vi "Kaelus PIM Set Stimulus.vi"(4 "Force? (f)":bool, 6 "Legacy (f)?":bool, 7 "TestSetDef":T1={"General"={"ID"=0, "Model"="", "Dual Port?"=FALSE, "Options"="", "Options"={"E"=FALSE, "K"=FALSE, "H"=FALSE, "W"=FALSE, "F"=FALSE}, "Cal File"=path ""}, "Receiver"={"Fstart, MHz"=0.0, "Fstop MHz"=0.0, "Fstep MHz"=0.0, "IF, MHz"=0.0}, "RX Band"={"Fstart, MHz"=0.0, "Fstop MHz"=0.0}, "TX 1"={"Fstart, MHz"=0.0, "Fstop MHz"=0.0, "Pmax, dBm"=0.0, "Pstep, dB"=0.0}, "TX 2"={"Fstart, MHz"=0.0, "Fstop MHz"=0.0, "Pmax, dBm"=0.0, "Pstep, dB"=0.0}, "Low-side?"=TRUE}, 8 "error in (no error)":errorcluster, 11 "Stimulus":T2={"Carrier Frequencies"={"C1 Freq, MHz"=0.0, "C2 Freq, MHz"=0.0}, "Carrier Powers"={"C1 Power,dBm"=0.0, "C2 Power, dBm"=0.0}, "Measurement Parameters"={"IM Order"=0, "Averaging"=1, "Direction"=0, "Enable ALC?"=FALSE, "Enable SingleIM?"=FALSE, "Display Units"=enum."dBm", "VA Hold?"=FALSE, "DUT PORT"=enum."Port 1"}, "Measurement Setup"={"Meas Type"=enum."Time", "TXStep"=0}} {"Measurement Setup"."TXStep" items=[".2", ".4", "1.0", "2.0"]; "Measurement Parameters"."Direction" items=["Reverse", "Forward", "Auxiliary"]; "Measurement Parameters"."IM Order" items=["3rd", "5th", "7th", "9th", "11th", "13th", "15th", "17th", "19th", "21st", "23rd", "25th", "27th", "29th", "31st", "33rd"]; "Measurement Parameters"."Averaging" items=["None", "Minimum", "Normal", "High", "Maximum"]}) -> (0 "error out":errorcluster, 2 "getSample Supported?":bool, 3 "Meas Type":enum32{"Time", "Frequency"}(ring))   [LabVIEW 2011]
uses:
  PIM Stimulus.ctl
  PIM Cmd Params.ctl
  BPIMCore/HW IO/IMOrder.ctl
  BPIMCore/HW IO/HW Averaging.ctl
  BPIMCore/HW IO/MeasMode.ctl
  BPIMCore/Display/display_unit_format.ctl
  BPIMCore/HW IO/DUTport.ctl
  BPIMCore/HW IO/PIM Sweep Step Size.ctl
  BPIMCore/HW IO/Test Set Definition.ctl
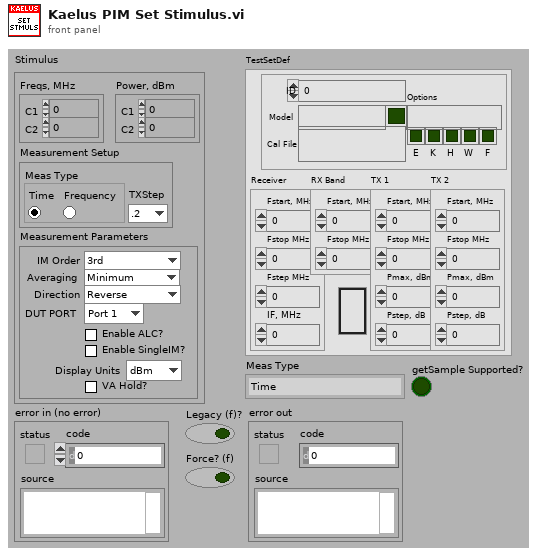
[diagram p1: front panel]
types:
  T1 = typedef "Test Set Definition.ctl" = cluster{"General":cluster{"ID":u32, "Model":string, "Dual Port?":bool, "Options":string, "Options":cluster{"E":bool, "K":bool, "H":bool, "W":bool, "F":bool}, "Cal File":path}, "Receiver":cluster{"Fstart, MHz":dbl, "Fstop MHz":dbl, "Fstep MHz":dbl, "IF, MHz":dbl}, "RX Band":cluster{"Fstart, MHz":dbl, "Fstop MHz":dbl}, "TX 1":cluster{"Fstart, MHz":dbl, "Fstop MHz":dbl, "Pmax, dBm":dbl, "Pstep, dB":dbl}, "TX 2":cluster{"Fstart, MHz":dbl, "Fstop MHz":dbl, "Pmax, dBm":dbl, "Pstep, dB":dbl}, "Low-side?":bool}
  T2 = typedef "PIM Stimulus.ctl" = cluster{"Carrier Frequencies":cluster{"C1 Freq, MHz":dbl, "C2 Freq, MHz":dbl}, "Carrier Powers":cluster{"C1 Power,dBm":dbl, "C2 Power, dBm":dbl}, "Measurement Parameters":T3, "Measurement Setup":cluster{"Meas Type":enum32{"Time", "Frequency"}, "TXStep":T9}}
  T3 = typedef "PIM Cmd Params.ctl" = cluster{"IM Order":T4, "Averaging":T5, "Direction":T6, "Enable ALC?":bool, "Enable SingleIM?":bool, "Display Units":T7, "VA Hold?":bool, "DUT PORT":T8}
  T4 = typedef "IMOrder.ctl" = u8
  T5 = typedef "HW Averaging.ctl" = u16
  T6 = typedef "MeasMode.ctl" = u16
  T7 = typedef "display_unit_format.ctl" = enum16{"dBm", "dBc"}
  T8 = typedef "DUTport.ctl" = enum16{"Port 1", "Port 2"}
  T9 = typedef "PIM Sweep Step Size.ctl" = u16
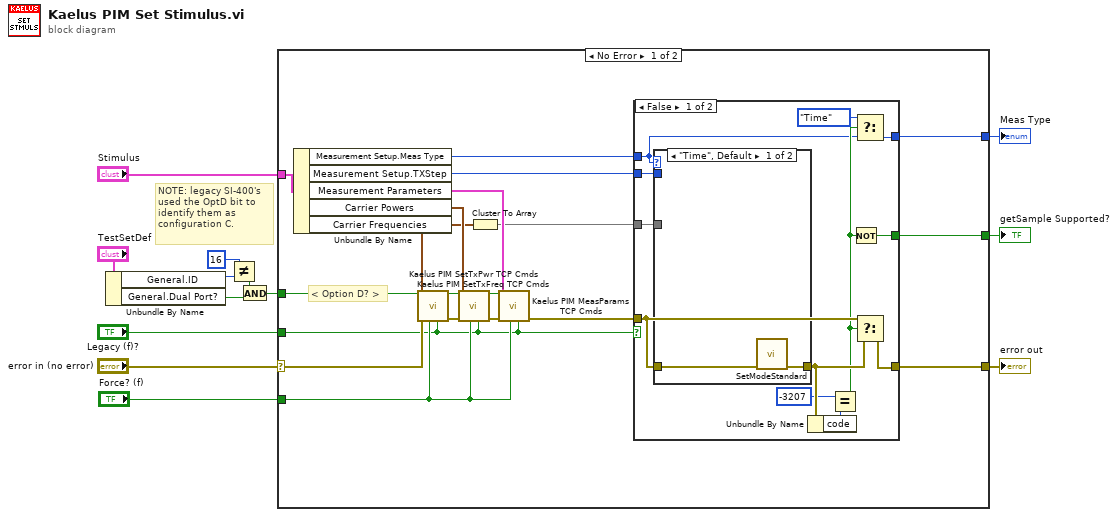
[diagram p0: block diagram]
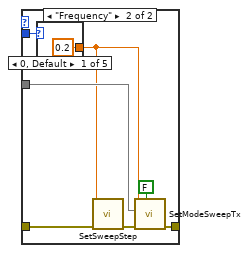
[diagram p2: hidden frame]
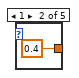
[diagram p3: hidden frame]
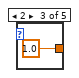
[diagram p4: hidden frame]
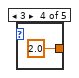
[diagram p5: hidden frame]
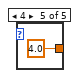
[diagram p6: hidden frame]
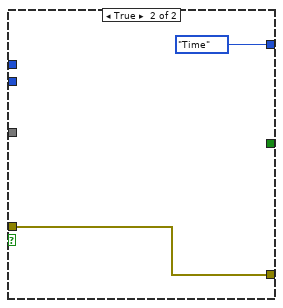
[diagram p7: hidden frame]
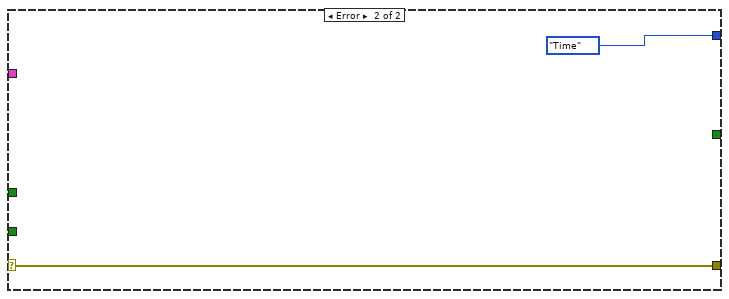
[diagram p8: hidden frame]
diagram:
  # "NOTE: legacy SI-400's\nused the OptD bit to \nidentify them as \nconfiguration C."
  n1 = Unbundle By Name("TestSetDef") -> ("General.ID"=w9:u32, "General.Dual Port?"=w6:bool)
  n2 = Not Equal?(x=16, y=w9) -> (x != y?=w7:bool)
  n3 = And(x=w7, y=w6) -> (x .and. y?=w5:bool)
  n4 = case shown="No Error" "error in (no error)" {
    selector: "error in (no error)" -> [w29 w60]
    tunnel: [w20 w60] -> w11
    tunnel: "Stimulus" -> [w30 _]
    tunnel: w5 -> [w26 _]
    tunnel: "Legacy (f)?" -> [w16 _]
    tunnel: "Force? (f)" -> [w24 _]
    tunnel: [w17 enum32{"Time", "Frequency"}."Time" ("Meas Type")] -> w2
    tunnel: [w15 _] -> w1
    frame No Error {
      # "< Option D? >"
      n5 = Unbundle By Name(w30) -> ("Measurement Setup.Meas Type"=w14:enum32{"Time", "Frequency"}, "Measurement Setup.TXStep"=w22:T9, "Measurement Parameters"=w25:T3, "Carrier Powers"=w23:cluster{"C1 Power,dBm":dbl, "C2 Power, dBm":dbl}, "Carrier Frequencies"=w19:cluster{"C1 Freq, MHz":dbl, "C2 Freq, MHz":dbl})
      n6 = call "Kaelus PIM SetTxFreq TCP Cmds.vi"("Legacy (f)?"=w16, "Force?"=w24, "error in"=w29, "Carrier Frequencies"=w19) -> ("error out"=w28:errorcluster)  [unwired: 7 out]
      n7 = call "Kaelus PIM SetTxPwr TCP Cmds.vi"("Legacy (f)?"=w16, "Force?"=w24, "error in"=w28, "Carrier Powers"=w23) -> ("error out"=w27:errorcluster)  [unwired: 7 out]
      n8 = Cluster To Array(cluster=w19) -> (array=w18:dbl[])
      n9 = call "Kaelus PIM MeasParams TCP Cmds.vi"("Option D?"=w26, "Legacy (f)?"=w16, "Force?"=w24, "error in"=w27, "Measurement Parameters"=w25) -> ("error out"=w21:errorcluster)  [unwired: 6 out]
      n10 = case shown="False" w16 {
        tunnel: w21 -> [w42 w57]
        tunnel: [w40 w57] -> w20
        tunnel: w18 -> [w39 _]
        tunnel: [w32 enum32{"Time", "Frequency"}."Time" ("Meas Type")] -> w17
        tunnel: [w37 _] -> w15
        tunnel: w22 -> [w33 _]
        tunnel: w14 -> [w31 _]
        frame False {
          n11 = case shown="\"Time\", Default" w31 {
            tunnel: w42 -> [w44 w49]
            tunnel: [w43 w51] -> w41
            tunnel: w39 -> [_ w47]
            tunnel: w33 -> [_ w46]
            frame "Time", Default {
              n12 = call "SetModeStandard.vi"("error in (no error)"=w44) -> ("error out"=w43:errorcluster)  [unwired: 10 in]
            }
            frame "Frequency" {
              n13 = case shown="0, Default" w46 {
                tunnel: [0.2 0.4 1.0 2.0 4.0] -> w45
                frame 0, Default {
                }
                frame 1 {
                }
                frame 2 {
                }
                frame 3 {
                }
                frame 4 {
                }
              }
              n14 = call "SetSweepStep.vi"("error in (no error)"=w49, "TX Freq Step Size"=w45) -> ("error out"=w48:errorcluster)  [unwired: 9 in]
              n15 = call "SetModeSweepTx.vi"("Full-Sweep?"=FALSE, "error in (no error)"=w48, "TxFrequencies"=w47, "Frequency Step"=w45) -> ("error out"=w51:errorcluster)  [unwired: 7 in]
            }
          }
          n16 = Unbundle By Name(w41) -> ("code"=w36:i32)
          n17 = Equal?(x=-3207, y=w36) -> (x = y?=w34:bool)
          n18 = Not(x=w34) -> (.not. x?=w37:bool)
          n19 = Select(t=enum32{"Time", "Frequency"}."Time" ("Measurement Setup.Meas Type"), s=w34, f=w31) -> (s? t:f=w32:enum32{"Time", "Frequency"})
          n20 = Select(t=w42, s=w34, f=w41) -> (s? t:f=w40:errorcluster)
        }
        frame True {
        }
      }
    }
    frame Error {
    }
  }
  "error out" <- w11
  "Meas Type" <- w2
  "getSample Supported?" <- w1
